vi "PID Output Rate Limiter Ext.vi"(0 "input (controller output)":dbl format="%.2f", 1 "reinitialize? (F)":bool, 5 "output old":dbl format="%.2f", 7 "output rate (EGU/s)":dbl=1.0 format="%.2f", 9 "Tick old":u32, 11 "dt (s)":dbl=-1.0 format="%.2f") -> (4 "output":dbl format="%.2f", 10 "Tick":u32, 15 "dt out (s)":dbl format="%.3f")   [LabVIEW 2019, in "control.lvlib"]
uses:
  control.lvlib
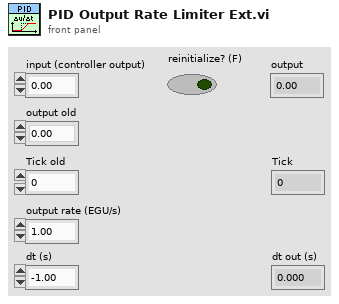
[diagram p1: front panel]
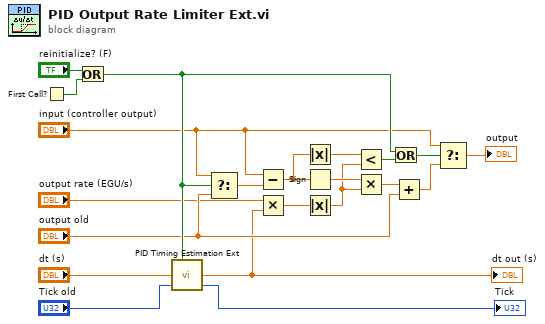
[diagram p0: block diagram]
diagram:
  n1 = First Call?() -> (First Call?: T/F=w20:bool)
  n2 = Or(x="reinitialize? (F)", y=w20) -> (x .or. y?=w19:bool)
  n3 = call "PID Timing Estimation Ext.vi"("R"=w19, "dt (s) in"="dt (s)", "Tick old"="Tick old") -> ("dt (s) out"=w1:dbl, "Tick"=→"Tick":u32)  [unwired: 5 in]
  "dt out (s)" <- w1
  n4 = Select(t="input (controller output)", s=w19, f="output old") -> (s? t:f=w9:dbl)
  n5 = Subtract(x="input (controller output)", y=w9) -> (x-y=w12:dbl)
  n6 = Multiply(x="output rate (EGU/s)", y=w1) -> (x*y=w14:dbl)
  n7 = Absolute Value(x=w12) -> (abs(x)=w7:dbl)
  n8 = Sign(1:w12) -> (0:w10:dbl)
  n9 = Absolute Value(x=w14) -> (abs(x)=w6:dbl)
  n10 = Less?(x=w7, y=w6) -> (x < y?=w13:bool)
  n11 = Multiply(x=w10, y=w6) -> (x*y=w8:dbl)
  n12 = Or(x=w19, y=w13) -> (x .or. y?=w5:bool)
  n13 = Add(x=w8, y="output old") -> (x+y=w11:dbl)
  n14 = Select(t="input (controller output)", s=w5, f=w11) -> (s? t:f=→"output":dbl)
